vi "Spread Out.vi"(11 "Impenetrable in":refnum<class "Impenetrable.lvclass">) -> (2 "64 out":refnum<class "Impenetrable.lvclass">, 3 "Impenetrable out":refnum<class "Impenetrable.lvclass">)   [LabVIEW 2015, in "Impenetrable.lvclass"]
uses:
  Impenetrable.lvclass
  Impenetrable.lvclass/Impenetrable.ctl
  Type.ctl
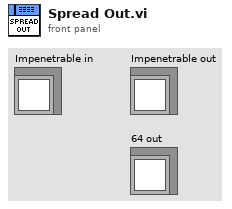
[diagram p1: front panel]
types:
  T1 = typedef "Common.lvlib/Position.ctl" = cluster{"Column":i32, "Row":i32}
  T2 = typedef "Impenetrable.lvclass/Type.ctl" = enum16{"Assassin", "Starter", "Line Starter", "ELine", "WLine", "StartPatrol", "WPatrol", "EPatrol", "WWall", "EWall", "Rain"}
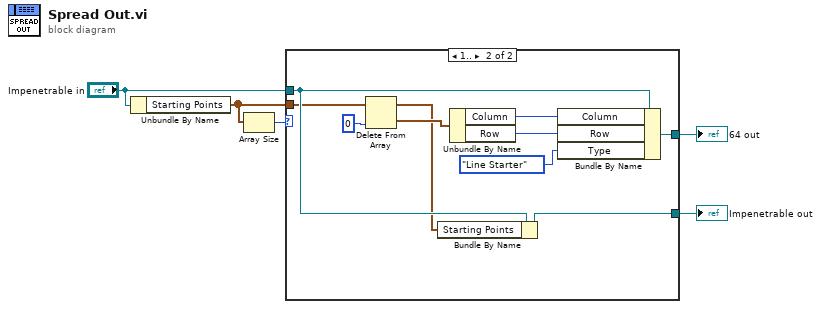
[diagram p0: block diagram]
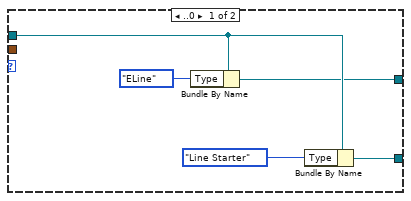
[diagram p2: hidden frame]
diagram:
  n1 = Unbundle By Name("Impenetrable in") -> ("Starting Points"=w5:T1[])
  n2 = Array Size(array=w5) -> (size(s)=w1:i32)
  n3 = case shown="1.." w1 {
    tunnel: "Impenetrable in" -> [w10 w20]
    tunnel: [w9 w12] -> w3
    tunnel: [w7 w19] -> w4
    tunnel: w5 -> [_ w18]
    frame ..0 {
      n4 = Bundle By Name(cluster=w10, "Type"=Type."ELine") -> (w7:refnum<class "Impenetrable.lvclass">)
      n5 = Bundle By Name(cluster=w10, "Type"=Type."Line Starter") -> (w9:refnum<class "Impenetrable.lvclass">)
    }
    frame 1.. {
      n6 = Delete From Array(array=w18, index=0) -> (deleted portion=w17:T1, array with subset deleted=w11:T1[])  [unwired: 1 in]
      n7 = Bundle By Name(cluster=w20, "Starting Points"=w11) -> (w12:refnum<class "Impenetrable.lvclass">)
      n8 = Unbundle By Name(w17) -> ("Column"=w13:i32, "Row"=w16:i32)
      n9 = Bundle By Name(cluster=w20, "Column"=w13, "Row"=w16, "Type"=Type."Line Starter") -> (w19:refnum<class "Impenetrable.lvclass">)
    }
  }
  "64 out" <- w4
  "Impenetrable out" <- w3
